vi "test_erp42mini.vi"() -> ()   [LabVIEW 2019]
panel:
  in  "AGV cfg":T1={"Port"="COM32", "speed limits"={"limit_linear-v"=0.5, "limit_angular-v"=0.7999999999999999}}
  in  "car_v":T2 {"speed_curr" format="%1_1g"; "Dir" scale=0.0..2.0; "Brake" scale=0.0..200.0; "Steer_set" scale=-2000.0..2000.0; "Acc_set" scale=0.0..100.0}
  in  "정지":bool
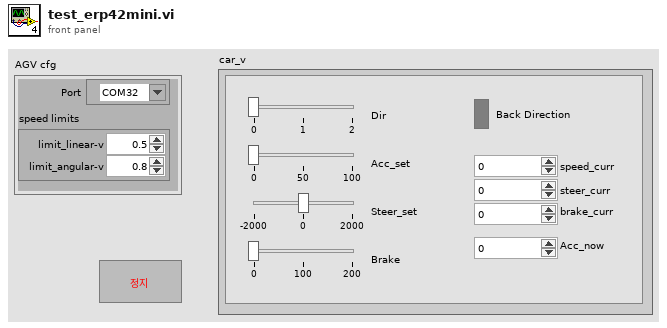
[diagram p1: front panel]
types:
  T1 = cluster{"Port":refnum<visa-resource-name>, "speed limits":cluster{"limit_linear-v":dbl, "limit_angular-v":dbl}}
  T2 = cluster{"Dir":u8, "Acc_set":u16, "Steer_set":i16, "Brake":i16, "Direction":bool, "speed_curr":dbl, "steer_curr":i16, "brake_curr":i16, "Acc_now":i16}
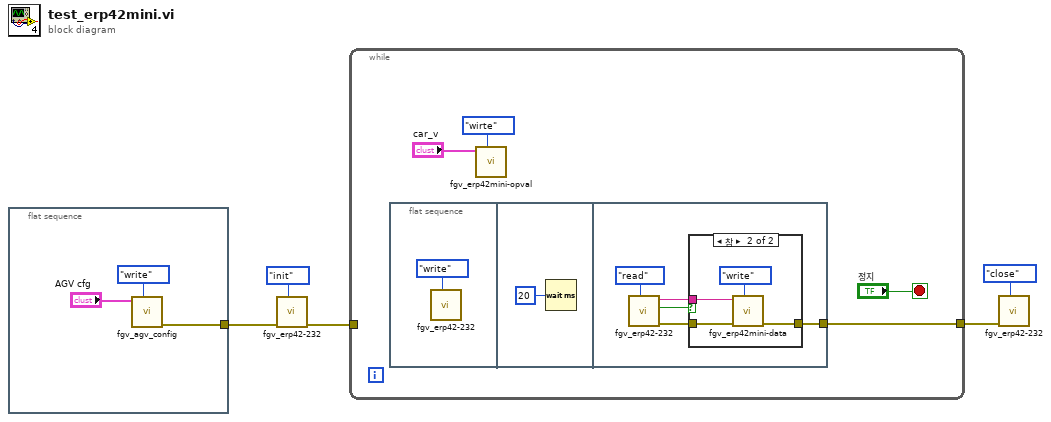
[diagram p0: block diagram]
diagram:
  n1 = flat-sequence {
    tunnel: [w6] -> w1
    frame #0 {
      n2 = call "fgv_agv_config.vi"("cmd"=enum16{"read", "write"}."write", "AGV cfg"="AGV cfg") -> ("error out"=w6:errorcluster)  [unwired: 8 in, 1 out]
    }
  }
  n3 = call "fgv_erp42-232.vi"("cmd"=enum16{"init", "read", "write", "close"}."init", "error in"=w1) -> ("error out"=w4:errorcluster)  [unwired: 7 in, 2 out]
  n4 = while {
    tunnel: w4 -> [_]
    tunnel: [w12] -> w2
    stop <- "정지" stop-if-true
    n5 = flat-sequence {
      tunnel: [w15] -> w12
      frame #0 {
        n6 = call "fgv_erp42-232.vi"("cmd"=enum16{"init", "read", "write", "close"}."write") -> ()  [unwired: 8 in, 3 out]
      }
      frame #1 {
        n7 = Wait (ms)(milliseconds to wait=u32 20 ("ms 배수")) -> ()  [unwired: 1 out]
      }
      frame #2 {
        n8 = call "fgv_erp42-232.vi"("cmd"=enum16{"init", "read", "write", "close"}."read") -> ("error out"=w16:errorcluster, "valid"=w18:bool, "read_buffer"=w17:string)  [unwired: 8 in]
        n9 = case shown="참" w18 {
          tunnel: w17 -> [_ w23]
          tunnel: w16 -> [w20 w22]
          tunnel: [w20 w21] -> w15
          frame False {
          }
          frame True {
            n10 = call "fgv_erp42mini-data.vi"("cmd"=enum16{"ini", "write", "read"}."write", "error in"=w22, "erp_read-data"=w23) -> ("error out"=w21:errorcluster)  [unwired: 7 in, 1 out]
          }
        }
      }
    }
    n11 = call "fgv_erp42mini-opval.vi"("cmd"=enum16{"ini", "read", "wirte"}."wirte", "car_v"="car_v") -> ()  [unwired: 9 in, 1 out]
  }
  n12 = call "fgv_erp42-232.vi"("cmd"=enum16{"init", "read", "write", "close"}."close", "error in"=w2) -> ()  [unwired: 7 in, 3 out]
